vi "TemperatureLogger.vi"() -> ()   [LabVIEW 2018]
uses:
  <vilib>/Analysis/NI_AALBase.lvlib
panel:
  in  "Temp input control":dbl(slide) scale=0.0..100.0
  out "Min Value":dbl format="%#_13g"
  out "Max Value":dbl format="%#_13g"
  out "Mean":dbl format="%#_13g"
  in  "stop":bool
  out "Current Data Point":dbl
  out "Current Data":dbl(slide) scale=0.0..100.0
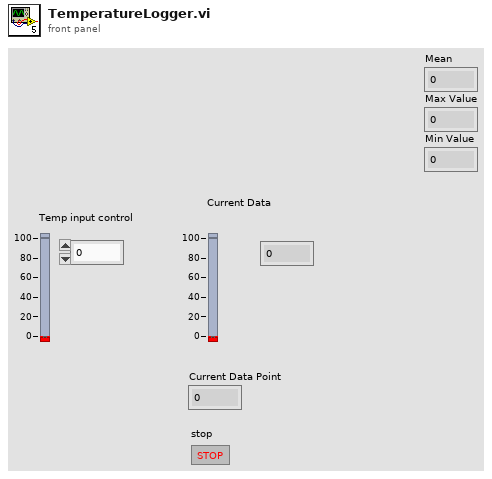
[diagram p1: front panel]
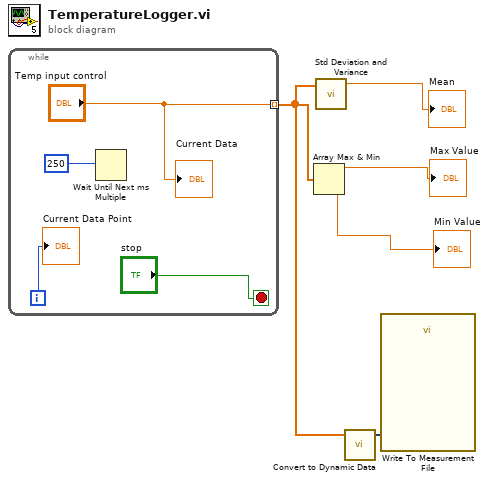
[diagram p0: block diagram]
diagram:
  n1 = while {
    tunnel: ["Temp input control"] -> w2 mode=indexing
    i -> [w8]
    stop <- "stop" stop-if-true
    n2 = Wait Until Next ms Multiple(millisecond multiple=250) -> ()  [unwired: 1 out]
    "Current Data" <- "Temp input control"
    "Current Data Point" <- w8
  }
  n3 = Array Max & Min(array=w2) -> (max value=→"Max Value":dbl, min value=→"Min Value":dbl)  [unwired: 2 out]
  n4 = call <vilib>:"Std Deviation and Variance.vi"("X"=w2) -> ("mean"=→"Mean":dbl)  [unwired: 1 in, 2 out]
  n5 = call "Convert to Dynamic Data"("Array"=w2) -> ("Dynamic Data Type"=w1:dynamicdata)  [unwired: 3 in]
  n6 = call "Write To Measurement File"("Signals"=w1) -> ()  [unwired: 16 in, 3 out]
